vi "Autonomous Independent.vi"() -> ()   [LabVIEW 2017]
doc: "This VI is called when autonomous begins, and will automatically be terminated when autonomous ends. You can carry out timed or sensor driven robot movement independently without needing to return to the caller."
uses:
  <vilib>/Rock Robotics/WPI/Solenoid/WPI_SolenoidValue.ctl
  <vilib>/Rock Robotics/Network Tables/NT Read String.vi
  <vilib>/Rock Robotics/WPI/Solenoid/WPI_SolenoidSetEnum.vi
panel:
  in  "Target Angle":dbl
  out "Refnum's Out":T1
  in  "Target Distance":dbl=15.0 format="%#_13g"
  out "Error Out":errorcluster
  in  "Error In":errorcluster
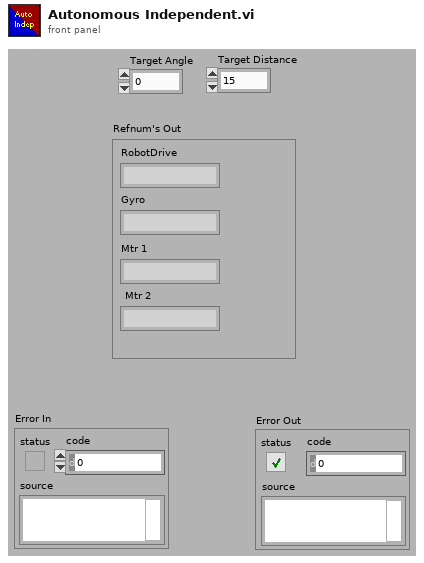
[diagram p1: front panel]
types:
  T1 = cluster{"RobotDrive":string, "Gyro":string, "Mtr 1":string, "Mtr 2":string}
  T2 = typedef "WPI_SolenoidValue.ctl" = enum16{"Off", "On", "Forward", "Reverse"}
  T3 = cluster{"Gyro":string, "Mtr 1":string, "Mtr 2":string}
  T4 = typedef "WPI_MotorControlDeviceRef.ctl" = cluster{"DeviceStatus":errorcluster, "Type":T5, "PWM":cluster{"PWM Channel":T6, "DeadBand":T7}, "CAN":cluster{"Device Number":u8, "SetOutput VI Ref":variant, "GetOutput VI Ref":variant, "Enable VI Ref":variant, "Disable VI Ref":variant, "Data":variant}, "Invert":bool, "DIO PWM":cluster{"PWM \"Enable\" Channel":T6, "DIOChannel":T8, "PWM Rate":dbl}}
  T5 = typedef "WPI_MotorControlType.ctl" = enum16{"PWM", "CAN", "DIO PWM"}
  T6 = typedef "FPGA_DIOPWMChannel.ctl" = enum8{"PWM 0", "PWM 1", "PWM 2", "PWM 3", "PWM 4", "PWM 5", "PWM 6", "PWM 7", "PWM 8", "PWM 9", "PWM MXP 0", "PWM MXP 1", "PWM MXP 2", "PWM MXP 3", "PWM MXP 4", "PWM MXP 5", "PWM MXP 6", "PWM MXP 7", "PWM MXP 8", "PWM MXP 9", "Invalid"}
  T7 = typedef "WPI_PWMDeadband.ctl" = cluster{"Name":string, "maxPositivePwm":i32, "minPositivePwm":i32, "centerPwm":i32, "maxNegativePwm":i32, "minNegativePwm":i32, "angularRange":u16}
  T8 = typedef "FPGA_DIOChannel.ctl" = enum8{"DIO 0", "DIO 1", "DIO 2", "DIO 3", "DIO 4", "DIO 5", "DIO 6", "DIO 7", "DIO 8", "DIO 9", "DIO MXP 0", "DIO MXP 1", "DIO MXP 2", "DIO MXP 3", "DIO MXP 4", "DIO MXP 5", "DIO MXP 6", "DIO MXP 7", "DIO MXP 8", "DIO MXP 9", "DIO MXP 10", "DIO MXP 11", "DIO MXP 12", "DIO MXP 13", "DIO MXP 14", "DIO MXP 15", "SPI Port CS1", "SPI Port CS2", "SPI Port CS3", "SPI Port MISO", "SPI Port MOSI", "Invalid"}
  T9 = typedef "WPI_GyroDevRef.ctl" = cluster{"DevStatus":errorcluster, "Analog Channel":T10, "Gain (VoltsPerDegree/Second)":dbl, "Gyro Type":enum16{"Analog", "XRS450"}, "Handle":i32, "SPI Bus":T11, "Device Found":bool, "Sample Rate":dbl, "Calibrate On Open":bool, "Offset":dbl}
  T10 = typedef "FPGA_AIChannel.ctl" = enum8{"AI 0", "AI 1", "AI 2", "AI 3", "AI MXP 0", "AI MXP 1", "AI MXP 2", "AI MXP 3", "Invalid"}
  T11 = typedef "spi_bus.ctl" = enum16{"SPI On-Board, CS0", "SPI On-Board, CS1", "SPI On-Board, CS2", "SPI On-Board, CS3", "SPI MXP", "Invalid"}
  T12 = typedef "WPI_SolenoidDevRef.ctl" = cluster{"DevStatus":errorcluster, "Pneumatics Control Module":u8, "Forward Solenoid Channel":T13, "Reverse Solenoid Channel":T13}
  T13 = typedef "WPI_SolenoidChannel.ctl" = enum8{"Solenoid 0", "Solenoid 1", "Solenoid 2", "Solenoid 3", "Solenoid 4", "Solenoid 5", "Solenoid 6", "Solenoid 7", "Invalid"}
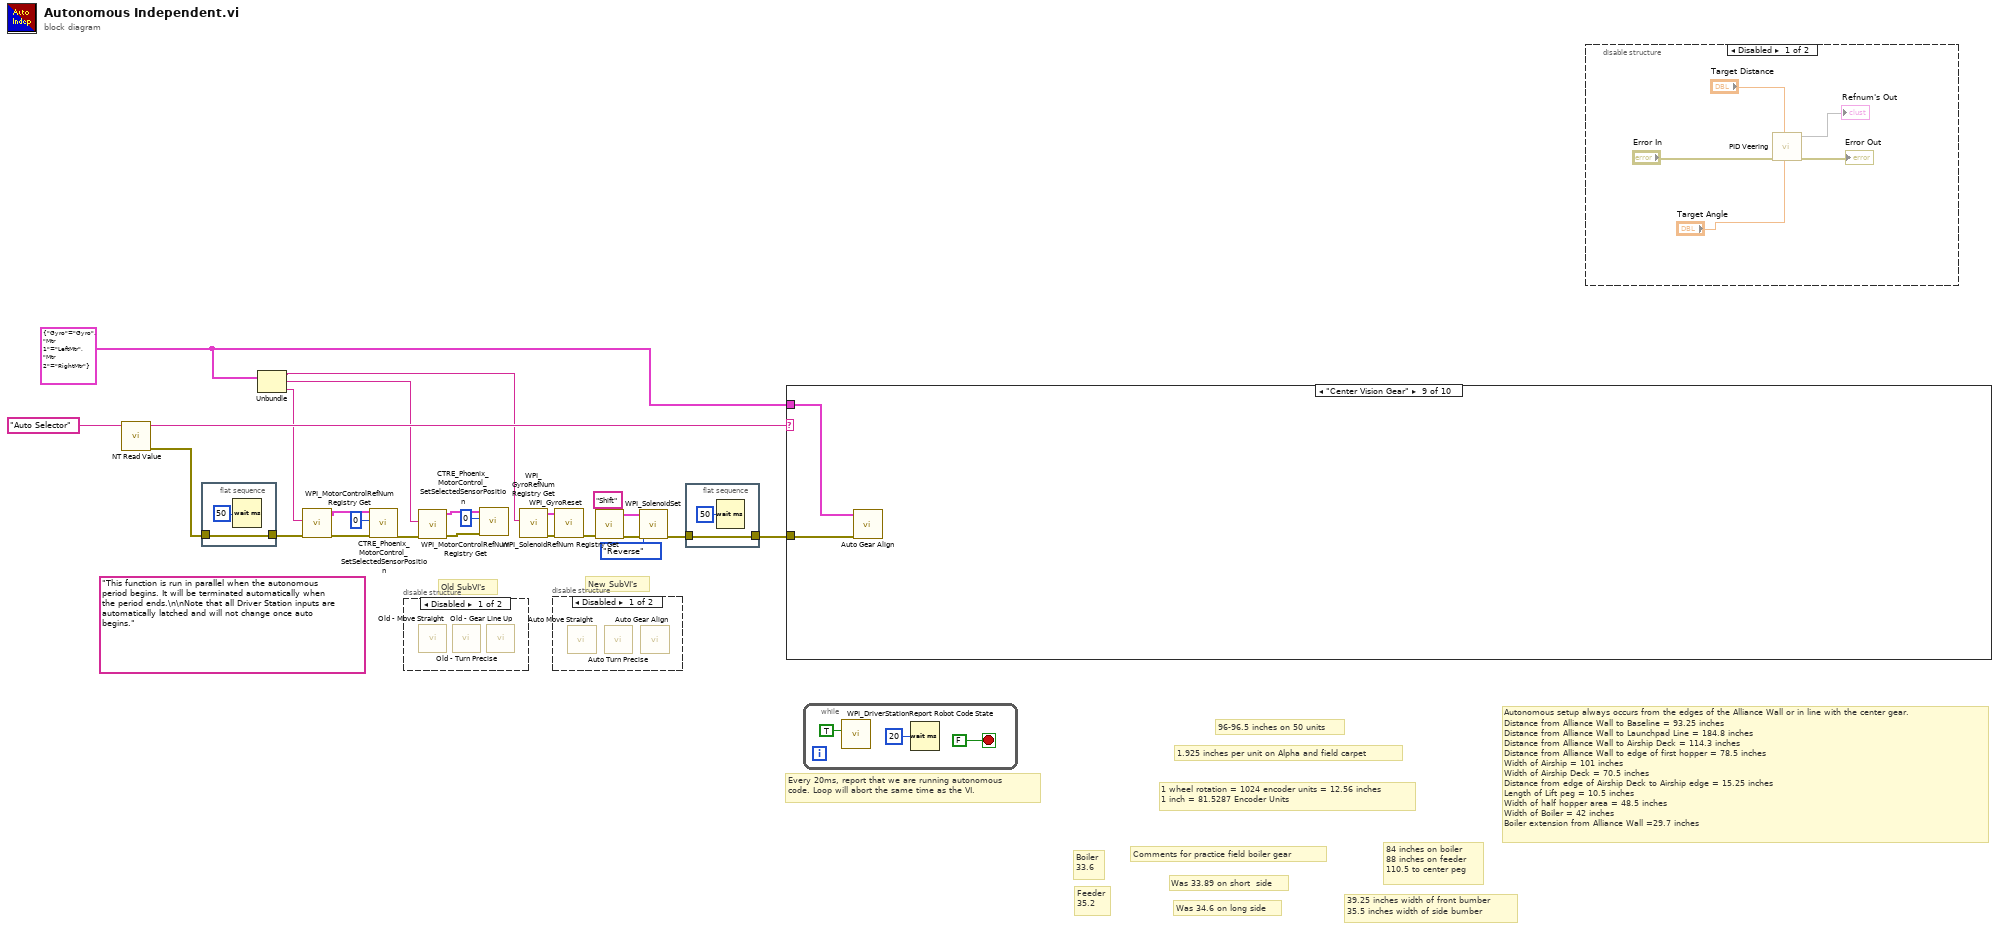
[diagram p0: block diagram]
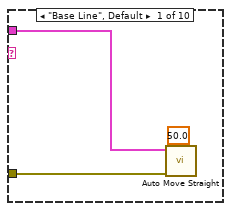
[diagram p3: hidden frame]
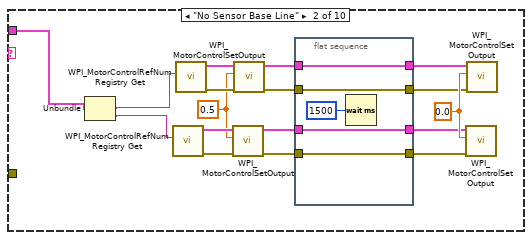
[diagram p4: hidden frame]
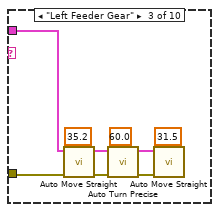
[diagram p5: hidden frame]
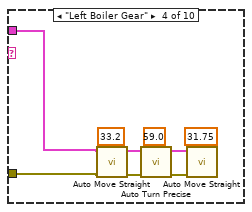
[diagram p6: hidden frame]
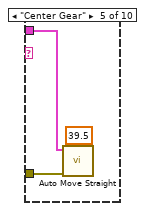
[diagram p7: hidden frame]
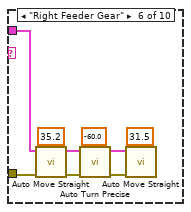
[diagram p8: hidden frame]
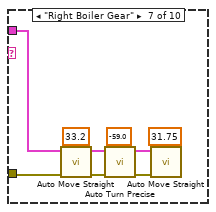
[diagram p9: hidden frame]
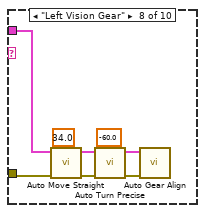
[diagram p10: hidden frame]
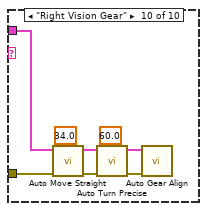
[diagram p11: hidden frame]
diagram:
  w11 = T3 {"Gyro"="Gyro", "Mtr 1"="LeftMtr", "Mtr 2"="RightMtr"} ("Refnum's")
  (unwired) "This function is run in parallel when the autonomous period begins. It will be terminated automatically when the period ends.\n\nNote that all Driver Station inputs are automatically latched and will not change once auto begins."
  # "39.25 inches width of front bumber\n35.5 inches width of side bumber"
  # "84 inches on boiler\n88 inches on feeder \n110.5 to center peg"
  # "1.925 inches per unit on Alpha and field carpet"
  # "96-96.5 inches on 50 units"
  # "Feeder\n35.2"
  # "Boiler\n33.6"
  # "Comments for practice field boiler gear"
  # "Was 34.6 on long side"
  # "Was 33.89 on short  side"
  # "New SubVI's"
  # "Old SubVI's"
  # "Autonomous setup always occurs from the edges of the Alliance Wall or in line with the center gear.\nDistance from Alliance Wall to Baseline = 93.25 inches\nDistance from Alliance Wall to Launchpad Line = 184.8 inches\nDistance from Alliance Wall to Airship Deck = 114.3 inches\nDistance from Alliance Wall to edge of first hopper = 78.5 inches\nWidth of Airship = 101 inches\nWidth of Airship Deck = 70.5 inches\nDistance from edge of Airship Deck to Airship edge = 15.25 inches\nLength of Lift peg = 10.5 inches\nWidth of half hopper area = 48.5 inches\nWidth of Boiler = 42 inches\nBoiler extension from Alliance Wall =29.7 inches"
  # "1 wheel rotation = 1024 encoder units = 12.56 inches\n1 inch = 81.5287 Encoder Units"
  # "Every 20ms, report that we are running autonomous\ncode. Loop will abort the same time as the VI."
  n1 = call-poly <vilib>:"NT Read Value.vi"("Name"="Auto Selector") -> ("error out"=w22:errorcluster, "String"=w23:string)  [unwired: 9 in]
  n2 = flat-sequence {
    tunnel: [w25] -> w14
    tunnel: w22 -> [w25]
    frame #0 {
      n3 = Wait (ms)(milliseconds to wait=u32 50) -> ()  [unwired: 1 out]
    }
  }
  n4 = Unbundle(w11) -> ("Gyro"=w10:string, "Mtr 1"=w9:string, "Mtr 2"=w8:string)
  n5 = call <vilib>:"WPI_MotorControlRefNum Registry Get.vi"("error in (no error)"=w14, "refnum name"=w8) -> ("error out"=w4:errorcluster, "MotorControlDevRef"=w3:T4)  [unwired: 8 in]
  n6 = call <vilib>:"CTRE_Phoenix_MotorControl_SetSelectedSensorPosition.vi"("error in (no error)"=w4, "New Sensor Position"=0, "PhoenixMotorControlDevRef"=w3) -> ("error out"=w5:errorcluster)  [unwired: 7 in, 1 out]
  n7 = disable-structure shown="Disabled" {
    frame Disabled {
      n8 = call "Old - Move Straight.vi"() -> ()  [unwired: 11 in, 1 out]
      n9 = call "Old - Turn Precise.vi"() -> ()  [unwired: 11 in, 1 out]
      n10 = call "Old - Gear Line Up.vi"() -> ()  [unwired: 11 in, 1 out]
    }
    frame Enabled {
    }
  }
  n11 = call <vilib>:"WPI_MotorControlRefNum Registry Get.vi"("error in (no error)"=w5, "refnum name"=w9) -> ("error out"=w6:errorcluster, "MotorControlDevRef"=w7:T4)  [unwired: 8 in]
  n12 = call <vilib>:"CTRE_Phoenix_MotorControl_SetSelectedSensorPosition.vi"("error in (no error)"=w6, "New Sensor Position"=0, "PhoenixMotorControlDevRef"=w7) -> ()  [unwired: 7 in, 2 out]
  n13 = call <vilib>:"WPI_GyroRefNum Registry Get.vi"("refnum name"=w10) -> ("error out"=w21:errorcluster, "GyroDevRef"=w20:T9)  [unwired: 9 in]
  n14 = disable-structure shown="Disabled" {
    frame Disabled {
      n15 = call "Auto Move Straight.vi"() -> ()  [unwired: 10 in, 2 out]
      n16 = call "Auto Turn Precise.vi"() -> ()  [unwired: 10 in, 2 out]
      n17 = call "Auto Gear Align.vi"() -> ()  [unwired: 10 in, 2 out]
    }
    frame Enabled {
    }
  }
  n18 = call <vilib>:"WPI_GyroReset.vi"("error in"=w21, "GyroDevRef"=w20) -> ("error out"=w15:errorcluster)  [unwired: 8 in, 1 out]
  n19 = call <vilib>:"WPI_SolenoidRefNum Registry Get.vi"("error in (no error)"=w15, "refnum name"="Shift") -> ("error out"=w19:errorcluster, "SolenoidDevRef"=w18:T12)  [unwired: 8 in]
  n20 = call-poly <vilib>:"WPI_SolenoidSet.vi"("error in (no error)"=w19, "Value"=WPI_SolenoidValue."Reverse", "SolenoidDevRef"=w18) -> ("error out"=w12:errorcluster)  [unwired: 7 in, 1 out]
  n21 = flat-sequence {
    tunnel: [w27] -> w13
    tunnel: w12 -> [w27]
    frame #0 {
      n22 = Wait (ms)(milliseconds to wait=u32 50) -> ()  [unwired: 1 out]
    }
  }
  n23 = case shown="\"Center Vision Gear\"" w23 {
    tunnel: w11 -> [w31 w34 w57 w65 w73 w75 w85 w93 w101 w103]
    tunnel: w13 -> [w30 _ w58 w66 w74 w76 w86 w94 w102 w104]
    frame "Base Line", Default {
      n24 = call "Auto Move Straight.vi"("Target Distance"=50.0, "Error In"=w30, "Refnum's In"=w31) -> ()  [unwired: 7 in, 2 out]
    }
    frame "No Sensor Base Line" {
      w43 = 0.0 ("Output")
      w44 = 0.5 ("Output")
      n25 = Unbundle(w34) -> ("Mtr 1"=w33:string, "Mtr 2"=w32:string)  [unwired: 1 out]
      n26 = call <vilib>:"WPI_MotorControlRefNum Registry Get.vi"("refnum name"=w32) -> ("error out"=w47:errorcluster, "MotorControlDevRef"=w48:T4)  [unwired: 9 in]
      n27 = call <vilib>:"WPI_MotorControlRefNum Registry Get.vi"("refnum name"=w33) -> ("error out"=w46:errorcluster, "MotorControlDevRef"=w45:T4)  [unwired: 9 in]
      n28 = call <vilib>:"WPI_MotorControlSetOutput.vi"("error in (no error)"=w47, "Output"=w44, "MotorControlDevRef"=w48) -> ("error out"=w37:errorcluster, "MotorControlDevRef"=w41:T4)  [unwired: 6 in, 1 out]
      n29 = call <vilib>:"WPI_MotorControlSetOutput.vi"("error in (no error)"=w46, "Output"=w44, "MotorControlDevRef"=w45) -> ("error out"=w36:errorcluster, "MotorControlDevRef"=w40:T4)  [unwired: 6 in, 1 out]
      n30 = flat-sequence {
        tunnel: [w52] -> w42
        tunnel: w41 -> [w52]
        tunnel: w40 -> [w51]
        tunnel: [w51] -> w39
        tunnel: [w50] -> w38
        tunnel: w37 -> [w50]
        tunnel: w36 -> [w49]
        tunnel: [w49] -> w35
        frame #0 {
          n31 = Wait (ms)(milliseconds to wait=u32 1500) -> ()  [unwired: 1 out]
        }
      }
      n32 = call <vilib>:"WPI_MotorControlSetOutput.vi"("error in (no error)"=w38, "Output"=w43, "MotorControlDevRef"=w42) -> ()  [unwired: 6 in, 3 out]
      n33 = call <vilib>:"WPI_MotorControlSetOutput.vi"("error in (no error)"=w35, "Output"=w43, "MotorControlDevRef"=w39) -> ()  [unwired: 6 in, 3 out]
    }
    frame "Left Feeder Gear" {
      n34 = call "Auto Move Straight.vi"("Target Distance"=35.2, "Error In"=w58, "Refnum's In"=w57) -> ("Error Out"=w62:errorcluster, "Refnum's Out"=w61:T3)  [unwired: 7 in]
      n35 = call "Auto Turn Precise.vi"("Target Distance"=60.0, "Error In"=w62, "Refnum's In"=w61) -> ("Error Out"=w60:errorcluster, "Refnum's Out"=w59:T3)  [unwired: 7 in]
      n36 = call "Auto Move Straight.vi"("Target Distance"=31.5, "Error In"=w60, "Refnum's In"=w59) -> ()  [unwired: 7 in, 2 out]
    }
    frame "Left Boiler Gear" {
      n37 = call "Auto Move Straight.vi"("Target Distance"=33.2, "Error In"=w66, "Refnum's In"=w65) -> ("Error Out"=w71:errorcluster, "Refnum's Out"=w70:T3)  [unwired: 7 in]
      n38 = call "Auto Turn Precise.vi"("Target Distance"=59.0, "Error In"=w71, "Refnum's In"=w70) -> ("Error Out"=w69:errorcluster, "Refnum's Out"=w68:T3)  [unwired: 7 in]
      n39 = call "Auto Move Straight.vi"("Target Distance"=31.75, "Error In"=w69, "Refnum's In"=w68) -> ()  [unwired: 7 in, 2 out]
    }
    frame "Center Gear" {
      n40 = call "Auto Move Straight.vi"("Target Distance"=39.5, "Error In"=w74, "Refnum's In"=w73) -> ()  [unwired: 7 in, 2 out]
    }
    frame "Right Feeder Gear" {
      n41 = call "Auto Move Straight.vi"("Target Distance"=35.2, "Error In"=w76, "Refnum's In"=w75) -> ("Error Out"=w77:errorcluster, "Refnum's Out"=w78:T3)  [unwired: 7 in]
      n42 = call "Auto Turn Precise.vi"("Target Distance"=-60.0, "Error In"=w77, "Refnum's In"=w78) -> ("Error Out"=w79:errorcluster, "Refnum's Out"=w80:T3)  [unwired: 7 in]
      n43 = call "Auto Move Straight.vi"("Target Distance"=31.5, "Error In"=w79, "Refnum's In"=w80) -> ()  [unwired: 7 in, 2 out]
    }
    frame "Right Boiler Gear" {
      n44 = call "Auto Move Straight.vi"("Target Distance"=33.2, "Error In"=w86, "Refnum's In"=w85) -> ("Error Out"=w87:errorcluster, "Refnum's Out"=w88:T3)  [unwired: 7 in]
      n45 = call "Auto Turn Precise.vi"("Target Distance"=-59.0, "Error In"=w87, "Refnum's In"=w88) -> ("Error Out"=w89:errorcluster, "Refnum's Out"=w90:T3)  [unwired: 7 in]
      n46 = call "Auto Move Straight.vi"("Target Distance"=31.75, "Error In"=w89, "Refnum's In"=w90) -> ()  [unwired: 7 in, 2 out]
    }
    frame "Left Vision Gear" {
      n47 = call "Auto Move Straight.vi"("Target Distance"=34.0, "Error In"=w94, "Refnum's In"=w93) -> ("Error Out"=w100:errorcluster, "Refnum's Out"=w99:T3)  [unwired: 7 in]
      n48 = call "Auto Turn Precise.vi"("Target Distance"=-60.0, "Error In"=w100, "Refnum's In"=w99) -> ("Error Out"=w96:errorcluster, "Refnum's Out"=w95:T3)  [unwired: 7 in]
      n49 = call "Auto Gear Align.vi"("Error In"=w96, "Refnum's In"=w95) -> ()  [unwired: 8 in, 2 out]
    }
    frame "Center Vision Gear" {
      n50 = call "Auto Gear Align.vi"("Error In"=w102, "Refnum's In"=w101) -> ()  [unwired: 8 in, 2 out]
    }
    frame "Right Vision Gear" {
      n51 = call "Auto Move Straight.vi"("Target Distance"=34.0, "Error In"=w104, "Refnum's In"=w103) -> ("Error Out"=w105:errorcluster, "Refnum's Out"=w106:T3)  [unwired: 7 in]
      n52 = call "Auto Turn Precise.vi"("Target Distance"=60.0, "Error In"=w105, "Refnum's In"=w106) -> ("Error Out"=w109:errorcluster, "Refnum's Out"=w110:T3)  [unwired: 7 in]
      n53 = call "Auto Gear Align.vi"("Error In"=w109, "Refnum's In"=w110) -> ()  [unwired: 8 in, 2 out]
    }
  }
  n54 = while {
    stop <- FALSE stop-if-true
    n55 = call <vilib>:"WPI_DriverStationReport Robot Code State.vi"("Autonomous"=TRUE) -> ()  [unwired: 10 in, 1 out]
    n56 = Wait (ms)(milliseconds to wait=u32 20) -> ()  [unwired: 1 out]
  }
  n57 = disable-structure shown="Disabled" {
    frame Disabled {
      n58 = call "PID Veering.vi"("Deviation"="Target Angle", "Current Distance"="Target Distance", "error in (no error)"="Error In") -> ("error out"=→"Error Out":errorcluster, 3:→"Refnum's Out")  [unwired: 7 in]
    }
    frame Enabled {
    }
  }
